vi "GENser Address Select.vi"(7 "GEN Addr":i16=-1, 8 "error":errorcluster, 11 "VISA":refnum<visa-resource-name>="COM1") -> (0 "error out":errorcluster, 2 "Last GEN Addr":i16=99, 3 "VISA out":refnum<visa-resource-name>)   [LabVIEW 2017]
doc: "This VI performs the addressing of any Genesys power supply for all the driver subVIs. If the \"GEN Addr\" control is wired and it's value has changed since the last call, this VI sends an \"ADR nn\" to open the new address.\n\nThis driver is called by each of higher-level drivers, so normally it is not used seperately in a LabView program."
panel:
  # "Send GEN Address"
  # "Lambda Genesys \n Serial Port\n  DC Power Supplies"
  # "Send new address command\n\"ADR nn\" if address has changed"
  # "( -1 = Default \n       = No Addr Change)"
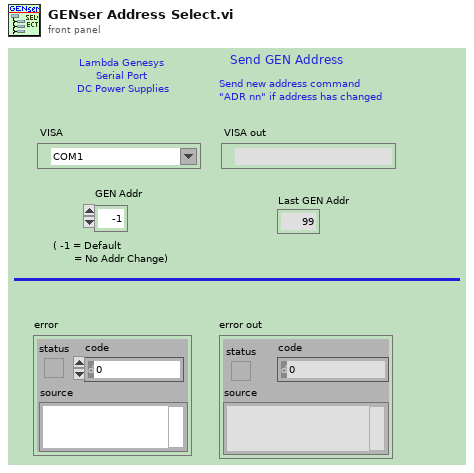
[diagram p1: front panel]
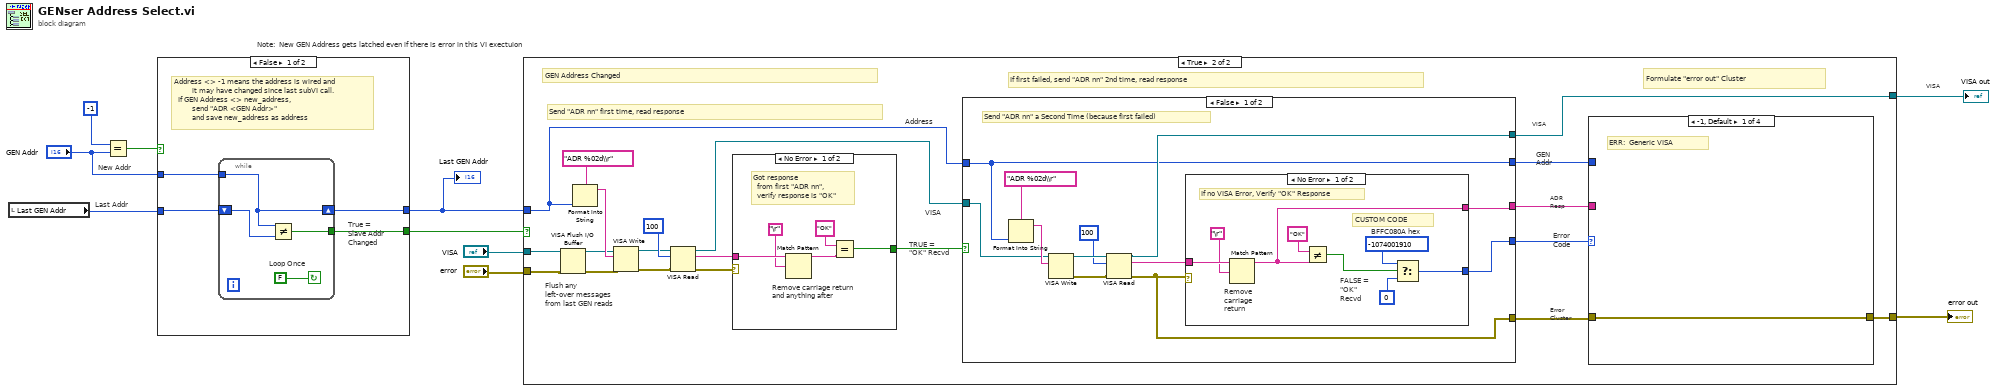
[diagram p0: block diagram]
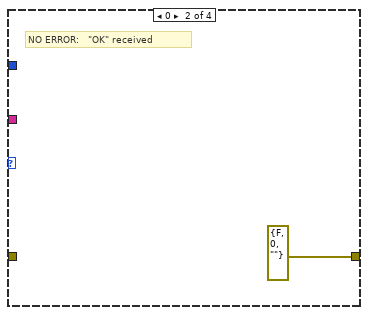
[diagram p3: hidden frame]
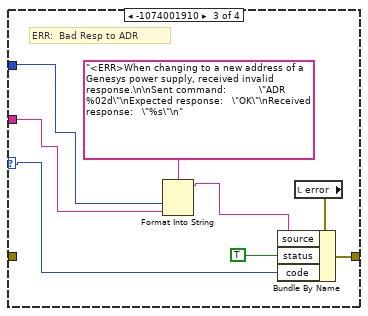
[diagram p4: hidden frame]
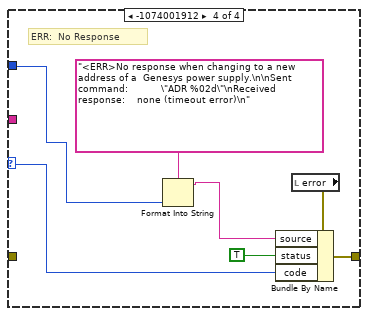
[diagram p5: hidden frame]
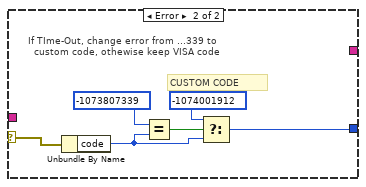
[diagram p6: hidden frame]
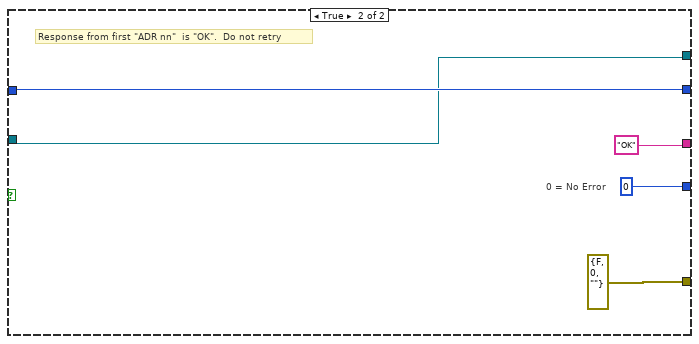
[diagram p7: hidden frame]
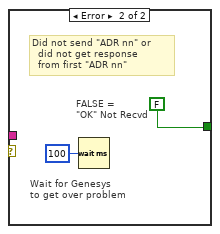
[diagram p8: hidden frame]
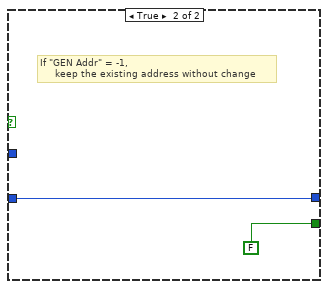
[diagram p9: hidden frame]
diagram:
  # "VISA"
  # "Note:  New GEN Address gets latched even if there is error in this VI exectuion"
  # "Last Addr"
  # "New Addr"
  n1 = local read "Last GEN Addr"() -> (w3:i16)
  n2 = Equal?(x=i16 -1 ("y"), y="GEN Addr") -> (x = y?=w10:bool)
  n3 = case shown="False" w10 {
    tunnel: "GEN Addr" -> [w14 _]
    tunnel: w3 -> [w13 w19]
    tunnel: [w12 FALSE] -> w7
    tunnel: [w11 w19] -> w1
    frame False {
      # "True = \nSlave Addr \nChanged"
      # "Address <> -1 means the address is wired and \n         it may have changed since last subVI call.  \n  If GEN Address <> new_address, \n         send \"ADR <GEN Addr>\"  \n         and save new_address as address"
      n4 = while {
        shift-right: [w15] -> w11
        shift-left: w13 -> [w17]
        tunnel: w14 -> [w15]
        tunnel: [w16] -> w12
        stop <- FALSE continue-if-true
        # "Loop Once"
        n5 = Not Equal?(x=w15, y=w17) -> (x != y?=w16:bool)
      }
    }
    frame True {
      # "If \"GEN Addr\" = -1,  \n     keep the existing address without change"
    }
  }
  "Last GEN Addr" <- w1
  n6 = case shown="True" w7 {
    tunnel: w1 -> [_ w30]
    tunnel: "VISA" -> [w21 w26]
    tunnel: "error" -> [w22 w24]
    tunnel: [w21 w29] -> w4
    tunnel: [w22 w27] -> w2
    frame False {
      # "Error In"
      # "VISA"
      # "VISA"
      # "Error In"
      # "Error In"
      # "VISA"
      # "GEN Address Did Not Change"
    }
    frame True {
      # "Flush any\nleft-over messages\nfrom last GEN reads"
      # "Formulate \"error out\" Cluster"
      # "VISA"
      # "GEN\nAddr"
      # "Error\nCluster"
      # "ADR \nResp"
      # "Error\nCode"
      # "GEN Address Changed"
      # "TRUE = \n\"OK\" Recvd"
      # "If first failed, send \"ADR nn\" 2nd time, read response"
      # "VISA"
      # "Address"
      # "Send \"ADR nn\" first time, read response"
      n7 = VISA Flush I/O Buffer(VISA resource name=w26, error in (no error)=w24) -> (VISA resource name out=w25:refnum<visa-resource-name>, error out=w23:errorcluster)  [unwired: 1 in]
      n8 = Format Into String(format string="ADR %02d\\r", w30) -> (resulting string=w39:string)  [unwired: 2 in, 1 out]
      n9 = VISA Write(VISA resource name=w25, write buffer=w39, error in (no error)=w23) -> (VISA resource name out=w40:refnum<visa-resource-name>, error out=w41:errorcluster)  [unwired: 1 out]
      n10 = VISA Read(VISA resource name=w40, byte count=u32 100 ("byte count (0)"), error in (no error)=w41) -> (VISA resource name out=w34:refnum<visa-resource-name>, read buffer=w36:string, error out=w37:errorcluster)  [unwired: 1 out]
      n11 = case shown="No Error" w37 {
        tunnel: w36 -> [w93 _]
        tunnel: [w92 FALSE] -> w35
        frame No Error {
          # "Remove carriage return\nand anything after"
          # "Got response \n  from first \"ADR nn\",  \n  verify response is \"OK\""
          n12 = Match Pattern(string=w93, regular expression="\r") -> (before substring=w95:string)  [unwired: 1 in, 3 out]
          n13 = Equal?(x="OK" ("regular expression"), y=w95) -> (x = y?=w92:bool)
        }
        frame Error {
          # "FALSE = \n\"OK\" Not Recvd"
          # "Wait for Genesys\nto get over problem"
          # "Did not send \"ADR nn\" or  \n  did not get response \n  from first \"ADR nn\""
          n14 = Wait (ms)(milliseconds to wait=u32 100) -> ()  [unwired: 1 out]
        }
      }
      n15 = case shown="False" w35 {
        tunnel: w34 -> [w66 w86]
        tunnel: w30 -> [w63 w90]
        tunnel: [w64 w86] -> w29
        tunnel: [w63 w90] -> w28
        tunnel: [w62 "OK"] -> w32
        tunnel: [w61 errorcluster {"status"=FALSE, "code"=0, "source"=""} ("error IO")] -> w33
        tunnel: [w60 0 ("code")] -> w31
        frame False {
          # "Send \"ADR nn\" a Second Time (because first failed)"
          n16 = Format Into String(format string="ADR %02d\\r", w63) -> (resulting string=w70:string)  [unwired: 2 in, 1 out]
          n17 = VISA Write(VISA resource name=w66, write buffer=w70) -> (VISA resource name out=w69:refnum<visa-resource-name>, error out=w68:errorcluster)  [unwired: 1 in, 1 out]
          n18 = VISA Read(VISA resource name=w69, byte count=u32 100 ("byte count (0)"), error in (no error)=w68) -> (VISA resource name out=w64:refnum<visa-resource-name>, read buffer=w65:string, error out=w61:errorcluster)  [unwired: 1 out]
          n19 = case shown="No Error" w61 {
            selector: w61 -> [_ w80]
            tunnel: w65 -> [w79 _]
            tunnel: [w78 _] -> w62
            tunnel: [w72 w81] -> w60
            frame No Error {
              # "If no VISA Error, Verify \"OK\" Response"
              # "CUSTOM CODE"
              # "BFFC080A hex"
              # "FALSE = \n\"OK\" \nRecvd"
              # "Remove \ncarriage\nreturn"
              n20 = Match Pattern(string=w79, regular expression="\r") -> (before substring=w78:string)  [unwired: 1 in, 3 out]
              n21 = Not Equal?(x="OK" ("regular expression"), y=w78) -> (x != y?=w73:bool)
              n22 = Select(t=-1074001910, s=w73, f=0) -> (s? t:f=w72:i32)
            }
            frame Error {
              # "If TIme-Out, change error from ...339 to  \n  custom code, othewise keep VISA code"
              # "CUSTOM CODE"
              n23 = Unbundle By Name(w80) -> ("code"=w84:i32)
              n24 = Equal?(x=-1073807339 ("code"), y=w84) -> (x = y?=w83:bool)
              n25 = Select(t=-1074001912 ("code"), s=w83, f=w84) -> (s? t:f=w81:i32)
            }
          }
        }
        frame True {
          # "0 = No Error"
          # "Response from first \"ADR nn\"  is \"OK\".  Do not retry"
        }
      }
      n26 = case shown="-1, Default" w31 {
        selector: w31 -> [_ _ w50 w56]
        tunnel: [w43 errorcluster {"status"=FALSE, "code"=0, "source"=""} ("error IO") w47 w57] -> w27
        tunnel: w33 -> [w43 _ _ _]
        tunnel: w32 -> [_ _ w49 _]
        tunnel: w28 -> [_ _ w48 w55]
        frame -1, Default {
          # "ERR:  Generic VISA"
        }
        frame 0 {
          # "NO ERROR:   \"OK\" received"
        }
        frame -1074001910 {
          # "ERR:  Bad Resp to ADR"
          n27 = Format Into String(format string="<ERR>When changing to a new address of a  Genesys power supply, received invalid response.\n\nSent command:           \"ADR %02d\"\nExpected response:   \"OK\"\nReceived response:   \"%s\"\n" ("Source (VI Name)"), w48, w49) -> (resulting string=w45:string)  [unwired: 2 in, 1 out]
          n28 = local read "error"() -> (w46:errorcluster)
          n29 = Bundle By Name(cluster=w46, "source"=w45, "status"=TRUE, "code"=w50) -> (w47:errorcluster)
        }
        frame -1074001912 {
          # "ERR:  No Response"
          n30 = Format Into String(format string="<ERR>No response when changing to a new address of a  Genesys power supply.\n\nSent command:           \"ADR %02d\"\nReceived response:    none (timeout error)\n" ("Source (VI Name)"), w55) -> (resulting string=w53:string)  [unwired: 2 in, 1 out]
          n31 = local read "error"() -> (w54:errorcluster)
          n32 = Bundle By Name(cluster=w54, "source"=w53, "status"=TRUE, "code"=w56) -> (w57:errorcluster)
        }
      }
    }
  }
  "error out" <- w2
  "VISA out" <- w4
